vi "Tracking_CreateFile.vi"(8 "error in":errorcluster, 10 "Settings in":T4={"Harware Configuration"={"Camera"="cam1", "Frames Per Second"=15, "Simulate Recording"=FALSE, "Simulated Recording Sample"=path "", "Timestamp Method"=enum."Camera Timestamp"}, "Base Recording Path"=path "", "Type Of Recording"="", "Recording Codec"="", "TrackingSettings"={"Max Radius"=0, "Threshold"=160.0, "ROI"={"Left"=0, "Top"=0, "Right"=0, "Bottom"=0, "Rotation"=0.0}}, "Calibration"={"Pixel Width (X)"=1.0, "Pixel Height (Y)"=1.0}, "Broadcast Length"=0} {"Broadcast Length" min=0; "TrackingSettings"."ROI"."Rotation" format="%.2f"; "TrackingSettings"."ROI"."Left" scale=0.0..1024.0; "TrackingSettings"."ROI"."Right" scale=0.0..1024.0; "TrackingSettings"."Threshold" scale=0.0..255.0}, 11 "Recording Data":T1) -> (0 "error out":errorcluster, 3 "Recording Data 2":T1)   [LabVIEW 2017, in "ImageAcquisitionLibrary.lvlib"]
uses:
  ImageAcquisitionLibrary.lvlib
  Settings/Settings.ctl
  <vilib>/userdefined/High Color/IMAQdx.ctl
  TrackingSettings.ctl
  Settings/Calibration.ctl
  Recording/RecordingData.ctl
  <vilib>/vision/Image Controls.llb/IMAQ Image.ctl
  <vilib>/vision/Avi.llb/IMAQ AVI2 Refnum.ctl
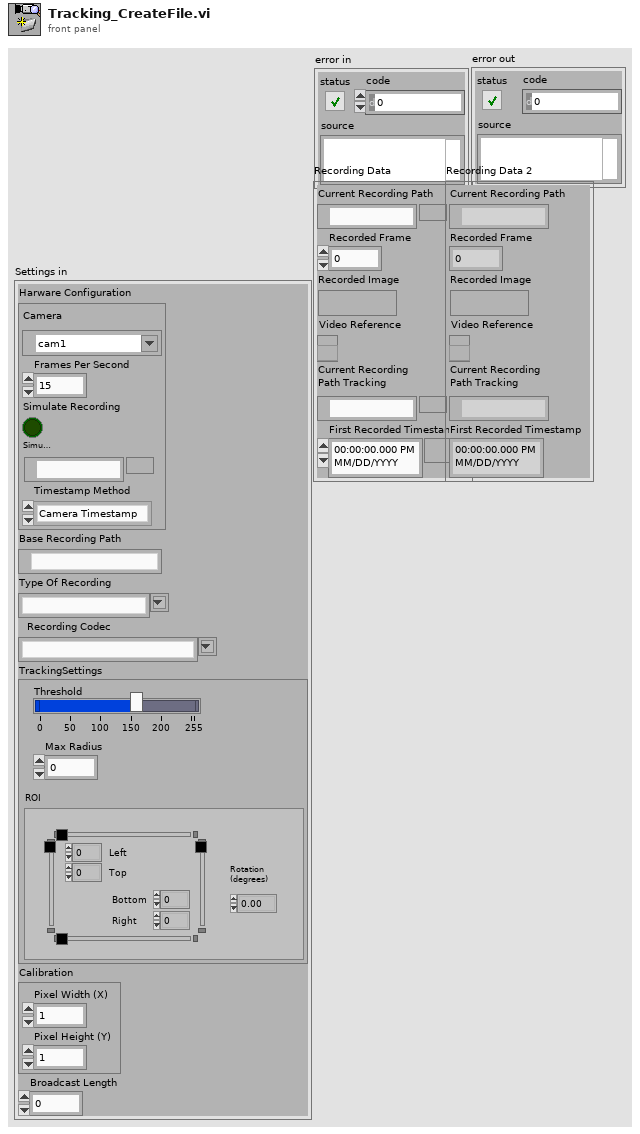
[diagram p1: front panel]
types:
  T1 = typedef "ImageAcquisitionLibrary.lvlib/RecordingData.ctl" = cluster{"Current Recording Path":path, "Recorded Frame":i32, "Recorded Image":T2, "Video Reference":T3, "Current Recording \nPath Tracking":path, "First Recorded Timestamp":timestamp}
  T2 = typedef "IMAQ Image.ctl" = refnum<image>
  T3 = typedef "IMAQ AVI2 Refnum.ctl" = refnum<k20>
  T4 = typedef "ImageAcquisitionLibrary.lvlib/Settings.ctl" = cluster{"Harware Configuration":cluster{"Camera":T5, "Frames Per Second":u32, "Simulate Recording":bool, "Simulated Recording Sample":path, "Timestamp Method":enum16{"System Timestamp", "Camera Timestamp", "IMAQdx Timestamp"}}, "Base Recording Path":path, "Type Of Recording":string, "Recording Codec":string, "TrackingSettings":T6, "Calibration":T8, "Broadcast Length":i32}
  T5 = typedef "IMAQdx.ctl" = refnum<k21>
  T6 = typedef "ImageAcquisitionLibrary.lvlib/TrackingSettings.ctl" = cluster{"Max Radius":i32, "Threshold":sgl, "ROI":T7}
  T7 = typedef "IMAQ Rectangle" = cluster{"Left":i32, "Top":i32, "Right":i32, "Bottom":i32, "Rotation":dbl}
  T8 = typedef "ImageAcquisitionLibrary.lvlib/Calibration.ctl" = cluster{"Pixel Width (X)":dbl, "Pixel Height (Y)":dbl}
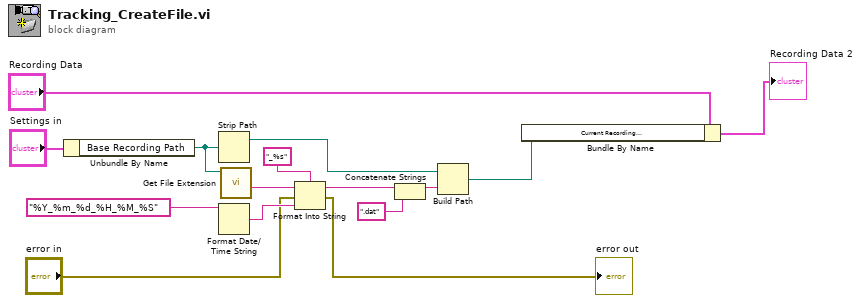
[diagram p0: block diagram]
diagram:
  n1 = Unbundle By Name("Settings in") -> ("Base Recording Path"=w10:path)
  n2 = Strip Path(path=w10) -> (stripped path=w15:path)  [unwired: 1 out]
  n3 = Format Date/Time String(time format string (%c)="%Y_%m_%d_%H_%M_%S") -> (date/time string=w13:string)  [unwired: 2 in]
  n4 = call <vilib>:"Get File Extension.vi"("file"=w10) -> ("filename without extension"=w8:string)  [unwired: 6 in, 4 out]
  n5 = Format Into String(format string="_%s", initial string=w8, error in="error in", w13) -> (resulting string=w7:string, error out=→"error out":errorcluster)
  n6 = Concatenate Strings(w7, ".dat") -> (w6:string)
  n7 = Build Path(base path=w15, name or relative path=w6) -> (appended path=w4:path)
  n8 = Bundle By Name(cluster="Recording Data", "Current Recording \nPath Tracking"=w4) -> (→"Recording Data 2":T1)
